vi "Create_Destination.vi"(8 "error in (no error)":errorcluster, 11 "AB_Dest_LLB in":refnum<class "AB_Dest_LLB.lvclass">) -> (0 "error out":errorcluster, 2 "directoriesCreated":path[](array[path]), 3 "AB_Dest_LLB out":refnum<class "AB_Dest_LLB.lvclass">)   [LabVIEW 2020, in "AB_Dest_LLB.lvclass"]
uses:
  <vilib>/AppBuilder/AB_Classes/Destination/Dest_LLB/AB_Dest_LLB.lvclass
  e:/builds/penguin/labview/branches/2020/dev/dist/vi.lib/AppBuilder/AB_Classes/Destination/AB_Destination.lvclass
  <vilib>/Utility/lvfile.llb/FT_FileTypes.ctl
  <vilib>/Utility/lvfile.llb/NI_FileType.lvlib
  <vilib>/AppBuilder/AB_Classes/Destination/AB_Destination.lvclass
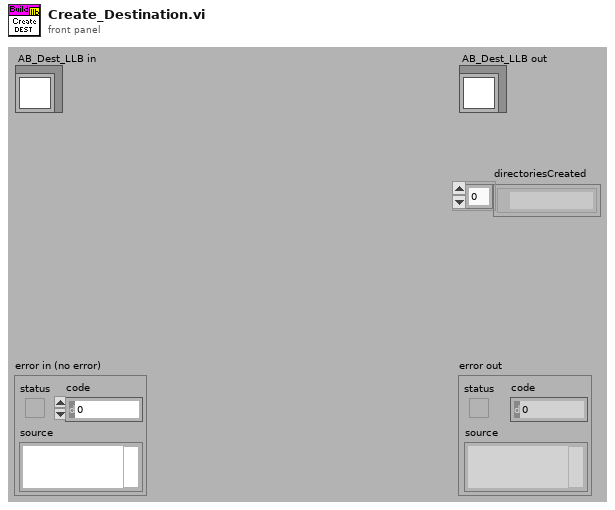
[diagram p1: front panel]
types:
  T1 = typedef "NI_FileType.lvlib/FT_FileTypes.ctl" = enum32{"Invalid file/path", "Unknown type", "Instrument", "Control", "Polymorphic VI", "Project", "Library", "LVClass", "XControl", "XNode", "CIN", "Run-time menu", "Palette menu", "LLB", "Shortcut", "Directory", "Class Private Data Control", "Statechart", "MathScript .m file", "Ladder Diagram", "LVLibp"}
  T2 = typedef "AB_Destination.ctl" = cluster{"destName":string, "path":path, "libraryName":string, "preserveHierarchy":bool, "eng_inBuild":bool, "eng_libraryReference":refnum<vi>, "eng_restictAddToNewLibrary":bool}
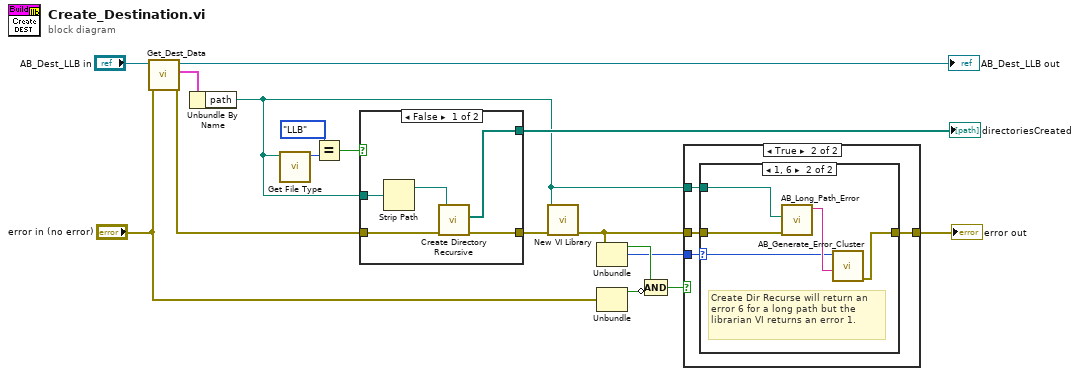
[diagram p0: block diagram]
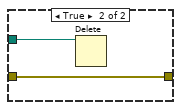
[diagram p4: hidden frame]
diagram:
  n1 = call <vilib>:"Get_Dest_Data.vi"("error in (no error)"="error in (no error)", "Class in"="AB_Dest_LLB in") -> ("error out"=w9:errorcluster, "destName"=w12:T2, "Class out"=→"AB_Dest_LLB out":refnum<class "AB_Dest_LLB.lvclass">)  [unwired: 7 in]
  n2 = Unbundle By Name(w12) -> ("path"=w4:path)
  n3 = call <vilib>:"Get File Type.vi"("path"=w4) -> ("file type"=w14:T1)  [unwired: 8 in, 2 out]
  n4 = Equal?(x=FT_FileTypes."LLB", y=w14) -> (x = y?=w13:bool)
  n5 = case shown="False" w13 {
    tunnel: w9 -> [w22 w24]
    tunnel: [w21 w24] -> w17
    tunnel: [w20 _] -> w16
    tunnel: w4 -> [w18 w23]
    frame False {
      n6 = Strip Path(path=w18) -> (stripped path=w19:path)  [unwired: 1 out]
      n7 = call <vilib>:"Create Directory Recursive.vi"("error in (no error)"=w22, "directory"=w19) -> ("error out"=w21:errorcluster, "directories created"=w20:path[])  [unwired: 3 in, 1 out]
    }
    frame True {
      n8 = Delete(path (use dialog)=w23) -> ()  [unwired: 4 in, 3 out]
    }
  }
  "directoriesCreated" <- w16
  n9 = call <vilib>:"New VI Library.vi"("error in (no error)"=w17, "VI library path in"=w4) -> ("error out"=w5:errorcluster)  [unwired: 8 in, 1 out]
  n10 = Unbundle(w5) -> ("status"=w6:bool, "code"=w1:i32)  [unwired: 1 out]
  n11 = Unbundle("error in (no error)") -> ("status"=w8:bool)  [unwired: 2 out]
  n12 = Compound Arithmetic op=AND(w6, invert w8) -> (w2:bool)
  n13 = case shown="True" w2 {
    tunnel: w5 -> [w25 w29]
    tunnel: w4 -> [_ w28]
    tunnel: [w25 w27] -> w3
    tunnel: w1 -> [_ w26]
    frame False {
    }
    frame True {
      n14 = case shown="1, 6" w26 {
        selector: w26 -> [_ w33]
        tunnel: w29 -> [w30 w31]
        tunnel: [w30 w32] -> w27
        tunnel: w28 -> [_ w35]
        frame Default {
        }
        frame 1, 6 {
          # "Create Dir Recurse will return an error 6 for a long path but the librarian VI returns an error 1."
          n15 = call <vilib>:"AB_Long_Path_Error.vi"("error in (no error)"=w31, "Path"=w35) -> ("error string out"=w34:string)  [unwired: 8 in, 1 out]
          n16 = call <vilib>:"AB_Generate_Error_Cluster.vi"("Additional Message"=w34, "Code"=w33) -> ("error out"=w32:errorcluster)  [unwired: 2 in, 7 out]
        }
      }
    }
  }
  "error out" <- w3
